vi "AudioIn Block Config Pane.vi"(6 "_SubPanelMessages":refnum<notifier>, 9 "_myEmbeddedToFrameEvent":T7, 10 "_myEmbedded.Exit":refnum<user-event>, 11 "-Property Bundle":cluster{"Name":string, "Value":variant}[](array[cluster])) -> (1 "_Connection Informations":T3, 2 "_Scripter Input":T9)   [LabVIEW 2021]
doc: "Reads values from one or more audio input channels on the NI myRIO. Use this Express VI to read multiple samples for each channel at one time."
uses:
  <vilib>/myRIO/Common/Express VI Framework/xctls/myRIO Channel List/myRIO Channel List.xctl
  <vilib>/myRIO/Common/Express VI Framework/typedefs/Config Pane to Framework Ref.ctl
  <vilib>/myRIO/Common/Express VI Framework/typedefs/Data Validate Ref.ctl
  <vilib>/myRIO/Common/Express VI Framework/typedefs/Scripter Input.ctl
  <vilib>/myRIO/Common/Express VI Framework/typedefs/WireThrough Terminal Names.ctl
  <vilib>/myRIO/Common/Express VI Framework/typedefs/Instrument Driver Method Descriptor Array.ctl
  <vilib>/myRIO/Common/Express VI Framework/typedefs/Instrument Driver Method Descriptor.ctl
  <vilib>/myRIO/Common/Express VI Framework/typedefs/Sub Panel Messages.ctl
  <vilib>/myRIO/Common/Express VI Framework/typedefs/Connection Informations.ctl
  <vilib>/myRIO/Common/Instrument Driver Framework/Utilities/typedefs/Channel Types.ctl
  <vilib>/myRIO/Common/Express VI Framework/vis/Express VI Framework Strings Global.vi
panel:
  in  "Sample Rate Unit":string="kHz"
  out "_learnMoreLatency":string="Gaps exist between sequential n samples acquisitions. Learn more"
  out "_learnMoreFrequency":string="Detailed information about valid sample rates for this Express VI.  Learn more"
  in  "_Validate":bool
  in  "Sample Rate:":dbl=1.0 caption="Sample rate:"
  in  "Samples to Read:":u32=1000 caption="Samples:" min=1 max=10000
  in  "Name:":string="Audio input (n samples)" caption="Node name:"
  in  "Selected Channel List":T1[](xcontrol)=[{"Channel Name"=0, "Channel Alias"="", "Remove Channel"=FALSE, "Index"=0}, {"Channel Name"=1, "Channel Alias"="", "Remove Channel"=FALSE, "Index"=1}]
  in  "_Default Alias String":string
  in  "_VI Default Name (Edit and make value default)":string="Audio input (n samples)"
  in  "_WireThrough Info (Edit and make value default)":T4={"WireThrough Top In"="AudioIn (N Samples) Ref In", "WireThrough Bottom In"="error in (no error)", "WireThrough Top Out"="AudioIn (N Samples) Ref Out", "WireThrough Bottom Out"="error out"}
  in  "_Template Array (Edit and make value default)":T5=[{"Function Name"="Smart Open", "VI Path"=path "<vilib>/myRIO/Instrument Drivers/Onboard IO/AudioIn Block/vis", "Script"=TRUE, "Inputs"=[{"name"="Channel Names", "value"=variant, "Config Pane Only"=TRUE, "Build Array"=FALSE, "Bundle Cluster"=FALSE, "Show Term"=FALSE, "alias"=[], "Required Input"=FALSE}], "Outputs"=[], "VI Class"=enum."Open", "Controls Refs[]"=[], "Inline"=FALSE}, {"Function Name"="Open", "VI Path"=path "<vilib>/myRIO/Instrument Drivers/Onboard IO/AudioIn Block/vis", "Script"=FALSE, "Inputs"=[{"name"="Channel Names", "value"=variant, "Config Pane Only"=TRUE, "Build Array"=FALSE, "Bundle Cluster"=FALSE, "Show Term"=FALSE, "alias"=[], "Required Input"=FALSE}], "Outputs"=[], "VI Class"=enum."Open", "Controls Refs[]"=[], "Inline"=FALSE}, {"Function Name"="Read", "VI Path"=path "<vilib>/myRIO/Instrument Drivers/Onboard IO/AudioIn Block/vis", "Script"=TRUE, "Inputs"=[{"name"="Number of Samples", "value"=variant, "Config Pane Only"=TRUE, "Build Array"=FALSE, "Bundle Cluster"=FALSE, "Show Term"=FALSE, "alias"=[], "Required Input"=TRUE}, {"name"="Sample Rate [Hz]", "value"=variant, "Config Pane Only"=TRUE, "Build Array"=FALSE, "Bundle Cluster"=FALSE, "Show Term"=FALSE, "alias"=[], "Required Input"=FALSE}], "Outputs"=[{"name"="Values", "value"=variant, "Show Term"=TRUE, "Index Array"=TRUE, "Unbundle Cluster"=FALSE, "alias"=[]}], "VI Class"=enum."Data", "Controls Refs[]"=[], "Inline"=FALSE}, {"Function Name"="Close", "VI Path"=path "<vilib>/myRIO/Instrument Drivers/Onboard IO/AudioIn Block/vis", "Script"=FALSE, "Inputs"=[], "Outputs"=[], "VI Class"=enum."Close", "Controls Refs[]"=[], "Inline"=FALSE}]
  in  "_Test Close":bool
  # "User Visible Area"
  # "NOTE: Tab Order has been set\nfor this Front Panel.\n1. Name: (string control)\n2. Add Channel (button)\n3. Selected Channel List (array)\n\nAll other controls are excluded \nfrom Tabbing order\n\nTo exlude a control from context\nhelp prefix its label text with a '-'"
  # "kHz"
  # "Gap:"
  # "Acquired signal"
  # "Missed signal"
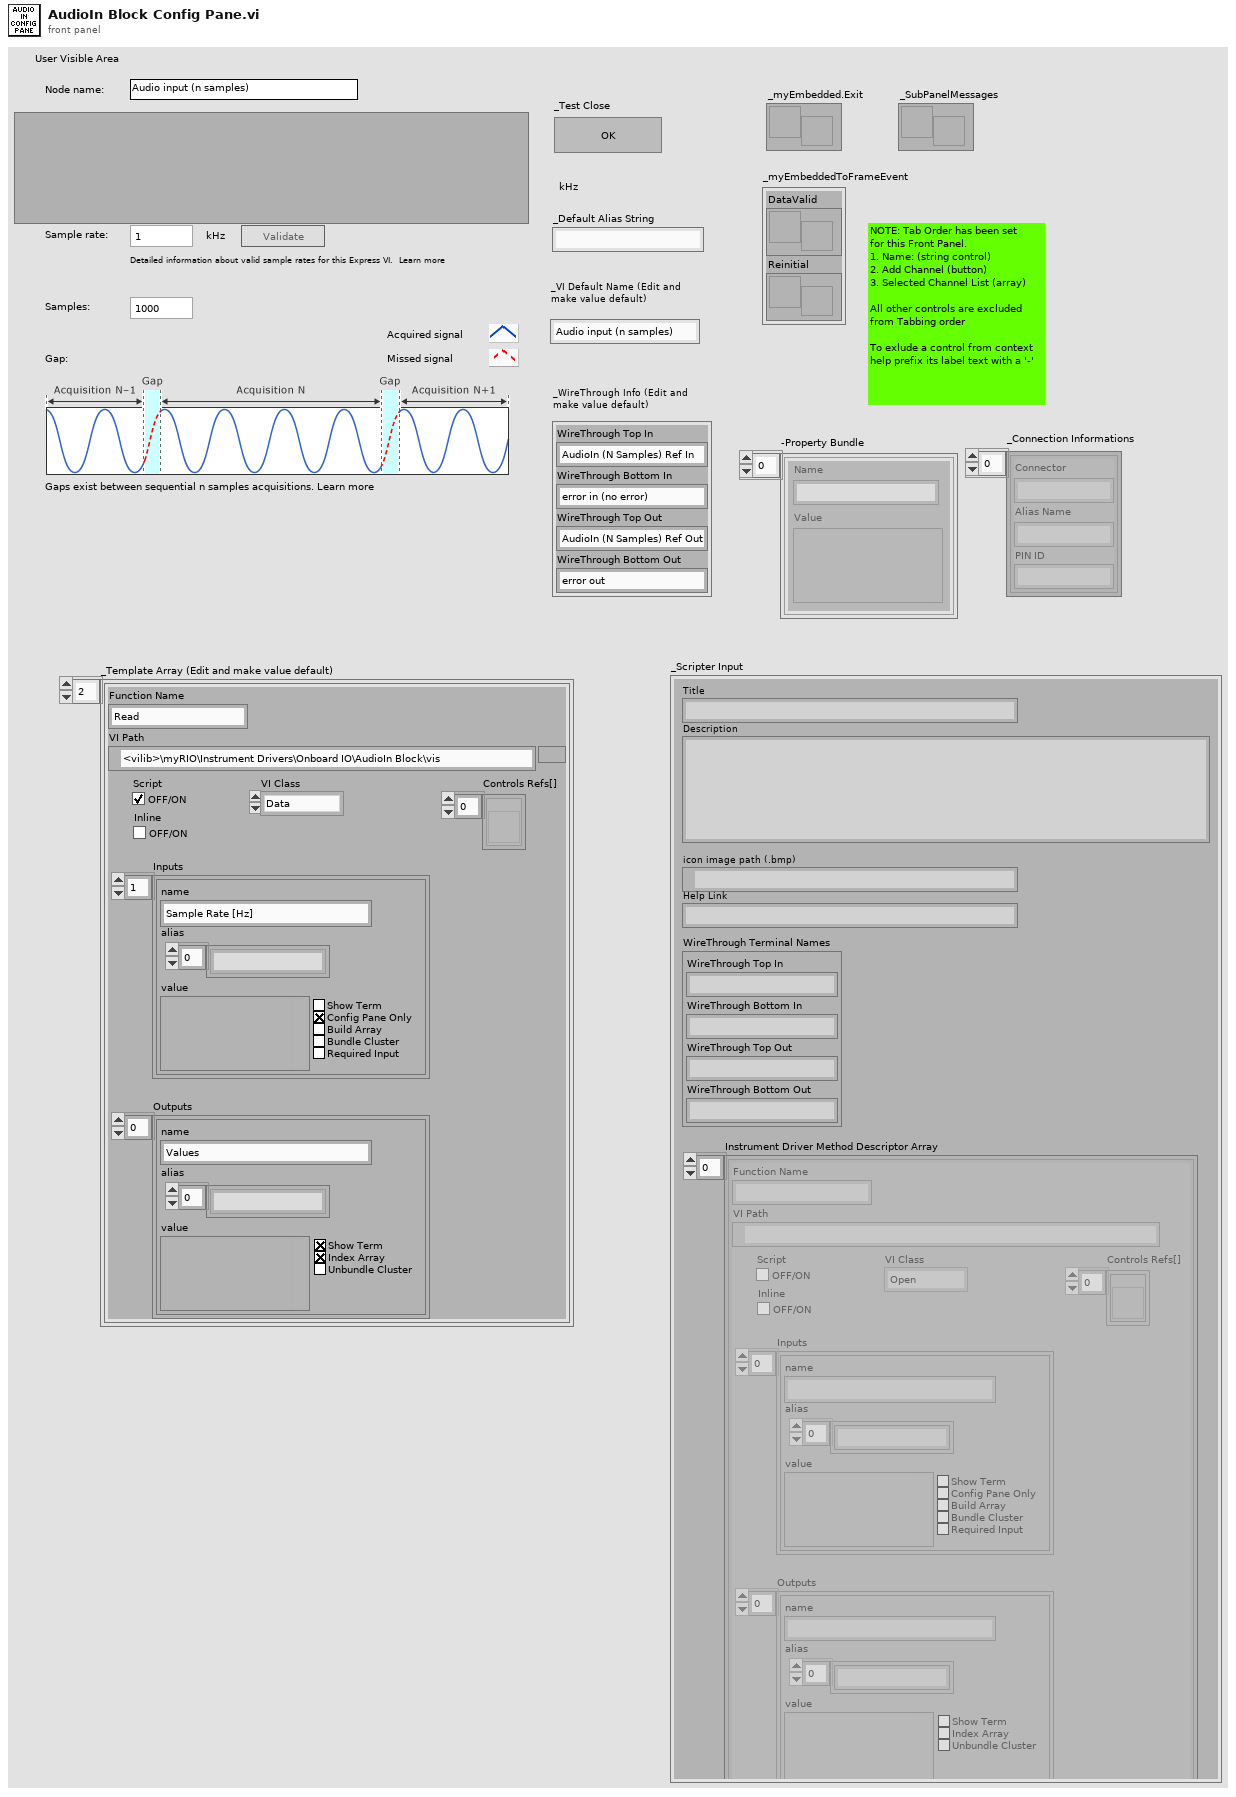
[diagram p1: front panel]
types:
  T1 = typedef "myRIO Channel List.xctl/Channel Data.ctl" = cluster{"Channel Name":u16, "Channel Alias":string, "Remove Channel":T2, "Index":i32}
  T2 = typedef "myRIO Channel List.xctl/Remove Channel.ctl" = bool
  T3 = typedef "Connection Informations.ctl" = cluster{"Connector":string, "Alias Name":string, "PIN ID":string}[]
  T4 = typedef "WireThrough Terminal Names.ctl" = cluster{"WireThrough Top In":string, "WireThrough Bottom In":string, "WireThrough Top Out":string, "WireThrough Bottom Out":string}
  T5 = typedef "Instrument Driver Method Descriptor Array.ctl" = T6[]
  T6 = typedef "Instrument Driver Method Descriptor.ctl" = cluster{"Function Name":string, "VI Path":path, "Script":bool, "Inputs":cluster{"name":string, "value":variant, "Config Pane Only":bool, "Build Array":bool, "Bundle Cluster":bool, "Show Term":bool, "alias":string[], "Required Input":bool}[], "Outputs":cluster{"name":string, "value":variant, "Show Term":bool, "Index Array":bool, "Unbundle Cluster":bool, "alias":string[]}[], "VI Class":enum16{"Open", "Configure", "Data", "Manage", "Close"}, "Controls Refs[]":refnum<vi>[], "Inline":bool}
  T7 = typedef "Config Pane to Framework Ref.ctl" = cluster{"DataValid":T8, "Reinitial":refnum<user-event>}
  T8 = typedef "Data Validate Ref.ctl" = refnum<user-event>
  T9 = typedef "Scripter Input.ctl" = cluster{"Title":string, "Description":string, "icon image path (.bmp)":path, "Help Link":string, "WireThrough Terminal Names":T4, "Instrument Driver Method Descriptor Array":T5}
  T10 = typedef "Channel Types.ctl" = enum32{"Unknown", "AI", "AO", "DIO - DI", "DIO", "DIO - DO", "I2C", "PWM", "Encoder", "SPI", "UART", "Accelerometer", "DIO - LED", "DIO - Button", "AI (N Samples)", "AudioIn (N Samples)", "AO (N Samples)", "AudioOut (N Samples)", "DI (N Samples)", "DO (N Samples)", "AI IRQ", "DI IRQ", "Timer IRQ", "RSL", "Relay", "CAN", "AI (Continuous)", "AO (Continuous)"}
  T11 = typedef "Channel Info.ctl" = cluster{"Channel Name":string, "Alias":string, "Used?":bool, "Not Support?":bool, "Property Bundle":cluster{"Name":string, "Value":variant}[]}
  T12 = typedef "Sub Panel Messages.ctl" = enum16{"Initialized"}
  T13 = enum8{"Enabled", "Disabled", "Disabled and Grayed Out"}
  T14 = cluster{"Connector":string, "Alias Name":string, "PIN ID":string}[]
  T15 = cluster{"name":string, "value":variant, "Config Pane Only":bool, "Build Array":bool, "Bundle Cluster":bool, "Show Term":bool, "alias":string[], "Required Input":bool}[]
  T16 = cluster{"name":string, "value":variant, "Config Pane Only":bool, "Build Array":bool, "Bundle Cluster":bool, "Show Term":bool, "alias":string[], "Required Input":bool}
  T17 = cluster{"name":string, "value":variant, "Show Term":bool, "Index Array":bool, "Unbundle Cluster":bool, "alias":string[]}[]
  T18 = cluster{"name":string, "value":variant, "Show Term":bool, "Index Array":bool, "Unbundle Cluster":bool, "alias":string[]}
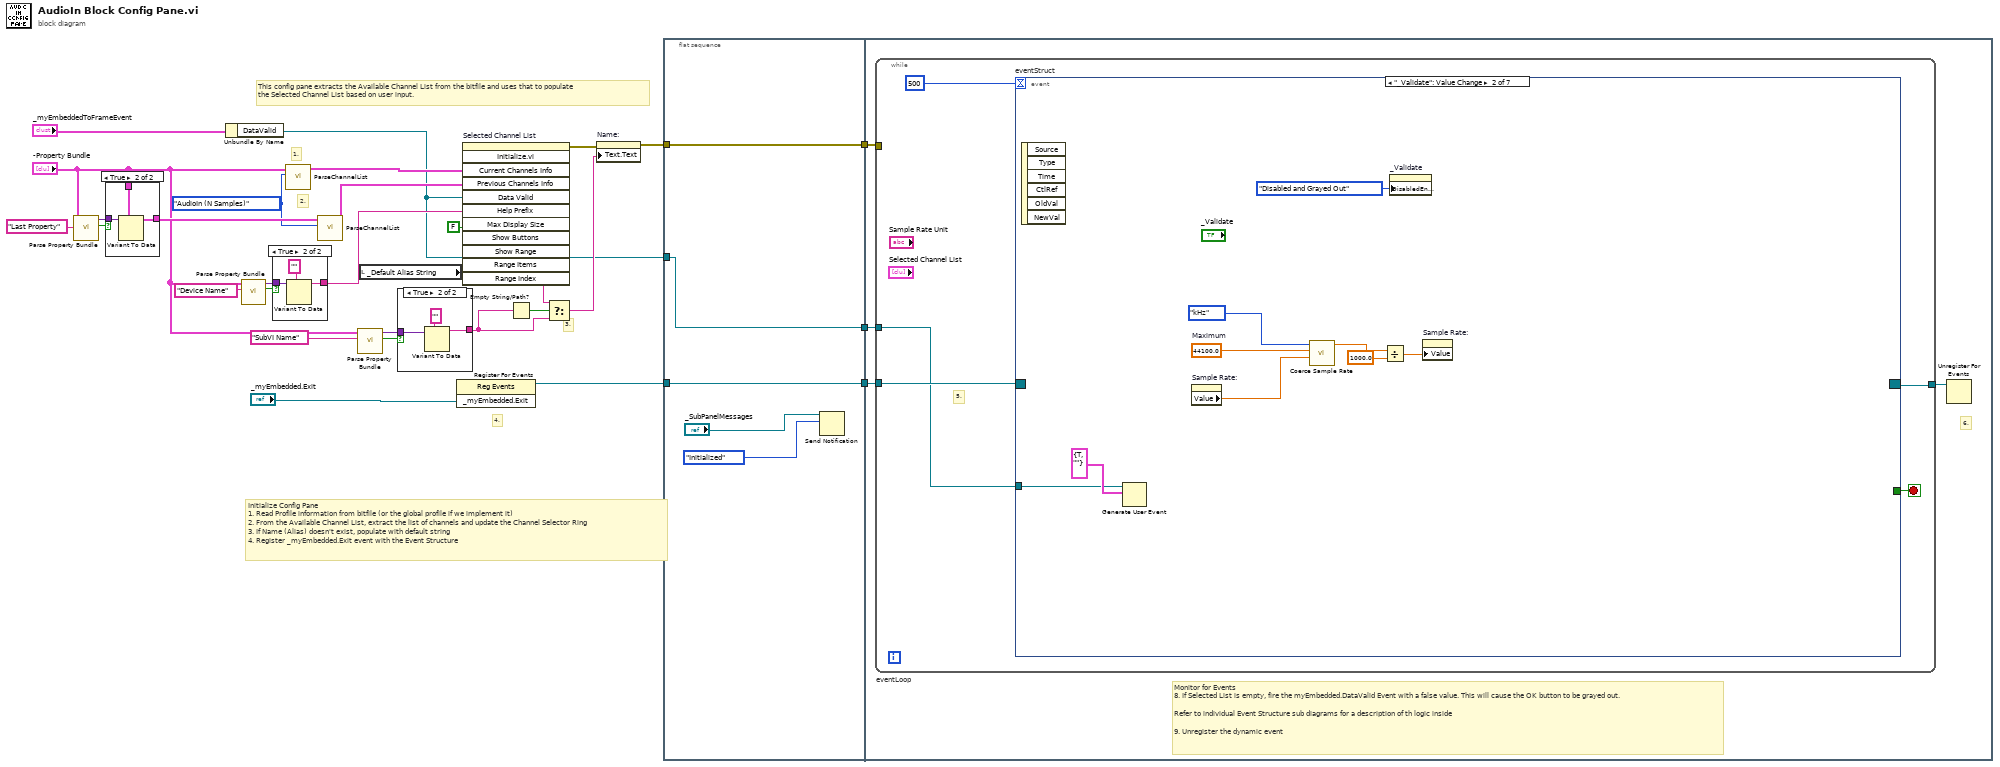
[diagram p0: block diagram]
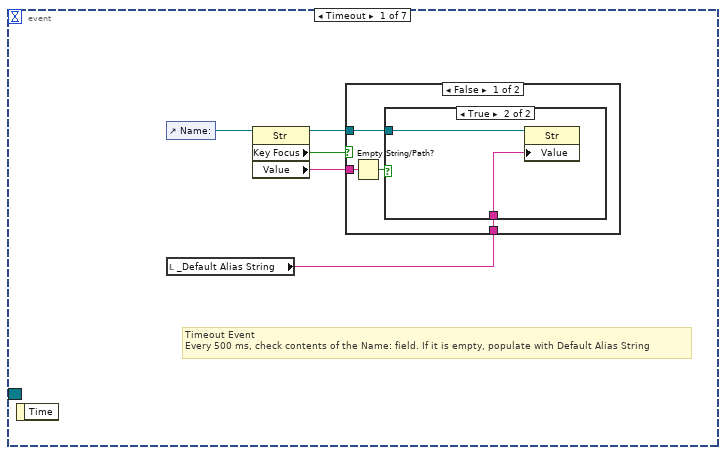
[diagram p2: hidden frame]
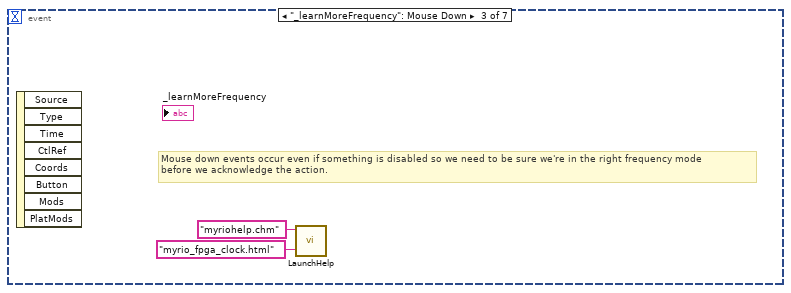
[diagram p5: hidden frame]
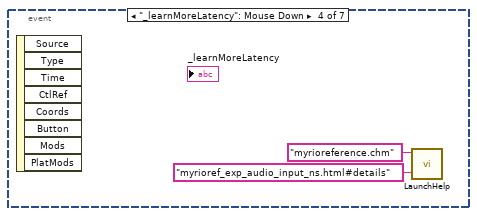
[diagram p6: hidden frame]
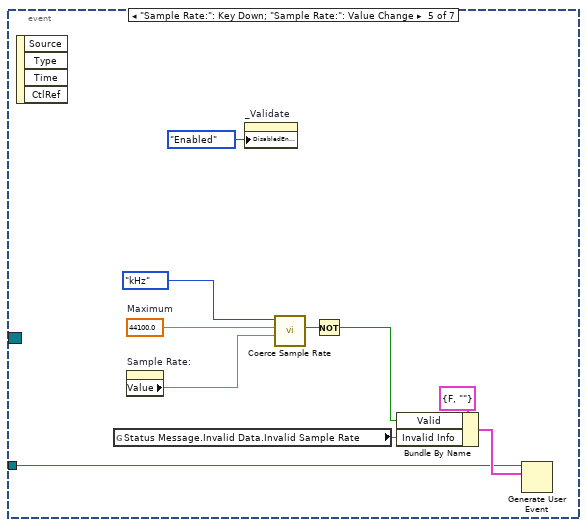
[diagram p7: hidden frame]
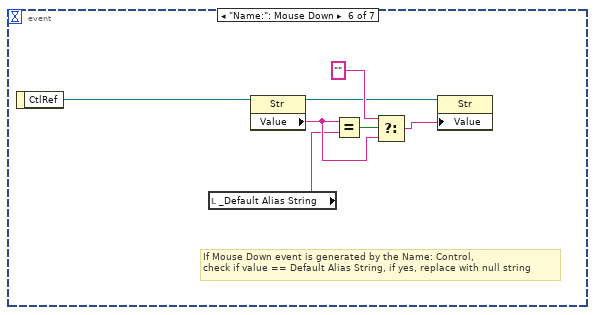
[diagram p8: hidden frame]
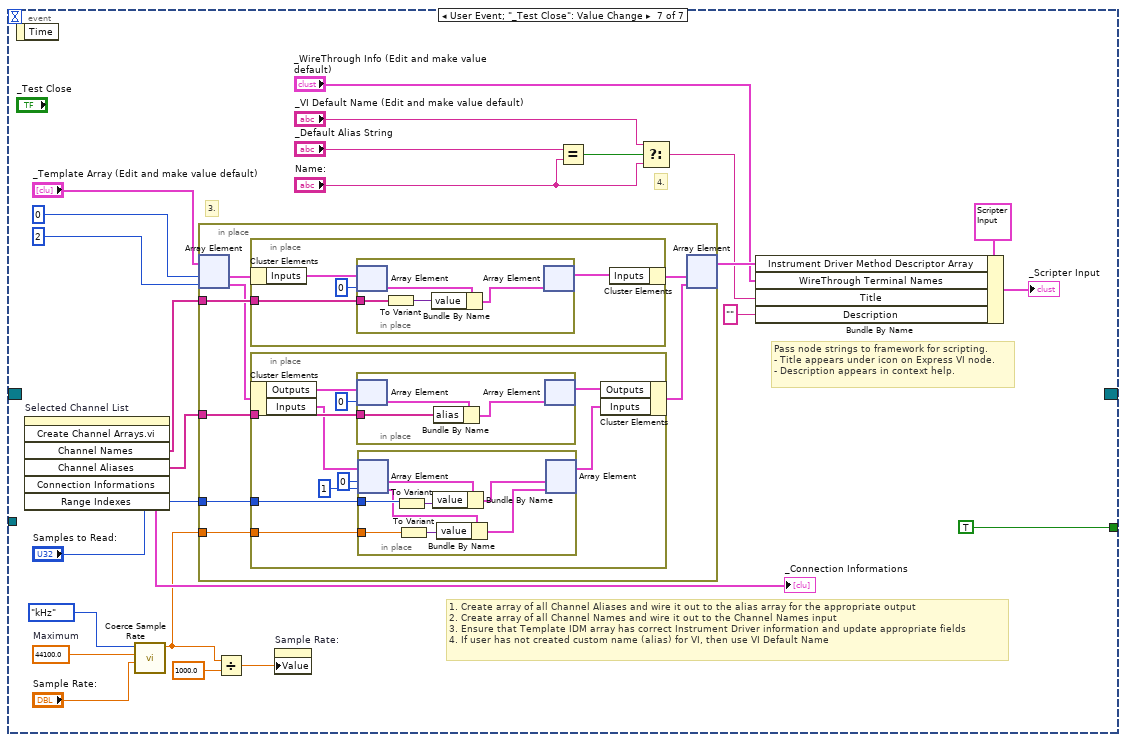
[diagram p9: hidden frame]
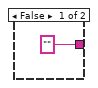
[diagram p12: hidden frame]
diagram:
  w12 = Channel_Types."AudioIn (N Samples)" ("Channel to Read")
  # "2."
  # "1."
  # "This config pane extracts the Available Channel List from the bitfile and uses that to populate\nthe Selected Channel List based on user input."
  # "4."
  # "3."
  # "Initialize Config Pane\n1. Read Profile information from bitfile (or the global profile if we implement it)\n2. From the Available Channel List, extract the list of channels and update the Channel Selector Ring\n3. If Name (Alias) doesn't exist, populate with default string\n4. Register _myEmbedded.Exit event with the Event Structure"
  n1 = call <vilib>:"Parse Property Bundle.vi"("Name"="Last Property", "Property Bundle"="-Property Bundle") -> ("Found?"=w15:bool, "Value"=w16:variant)  [unwired: 8 in]
  n2 = case shown="True" w15 {
    tunnel: w16 -> [_ w32]
    tunnel: [_ w31] -> w14
    tunnel: "-Property Bundle" -> [_ w30]
    frame False {
    }
    frame True {
      n3 = Variant To Data(type=w30, Variant=w32) -> (data=w31:cluster{"Name":string, "Value":variant}[])  [unwired: 1 in, 1 out]
    }
  }
  n4 = Unbundle By Name("_myEmbeddedToFrameEvent") -> ("DataValid"=w2:T8)
  n5 = call <vilib>:"Parse Property Bundle.vi"("Name"="Device Name", "Property Bundle"="-Property Bundle") -> ("Found?"=w9:bool, "Value"=w8:variant)  [unwired: 8 in]
  n6 = case shown="True" w9 {
    tunnel: w8 -> [_ w35]
    tunnel: [_ w34] -> w5
    frame False {
    }
    frame True {
      n7 = Variant To Data(type="", Variant=w35) -> (data=w34:string)  [unwired: 1 in, 1 out]
    }
  }
  n8 = call <vilib>:"ParseChannelList.vi"("Channel to Read"=w12, "_Property Bundle"="-Property Bundle") -> ("Channel List Out"=w19:T11[])  [unwired: 7 in, 2 out]
  n9 = call <vilib>:"ParseChannelList.vi"("Channel to Read"=w12, "_Property Bundle"=w14) -> ("Channel List Out"=w13:T11[])  [unwired: 7 in, 2 out]
  n10 = call <vilib>:"Parse Property Bundle.vi"("Name"="SubVI Name", "Property Bundle"="-Property Bundle") -> ("Found?"=w23:bool, "Value"=w24:variant)  [unwired: 8 in]
  n11 = local read "_Default Alias String"() -> (w18:string)
  n12 = case shown="True" w23 {
    tunnel: w24 -> [_ w39]
    tunnel: ["" ("Name") w37] -> w22
    frame False {
    }
    frame True {
      n13 = Variant To Data(type="" ("Name"), Variant=w39) -> (data=w37:string)  [unwired: 1 in, 1 out]
    }
  }
  n14 = register-events("_myEmbedded.Exit") -> (reference out=w21:refnum<event-registration>)  [unwired: 2 in, 1 out]
  n15 = invoke on="Selected Channel List" class="myRIO Channel List (strict)" method="Initialize.vi"("Current Channels Info"=w19, "Previous Channels Info"=w13, "Data Valid"=w2, "Help Prefix"=w5, "Show Buttons"=FALSE) -> (error out=w20:errorcluster)  [unwired: 7 in, 11 out]
  n16 = Empty String/Path?(string/path=w22) -> (empty?=w28:bool)
  n17 = Select(t=w18, s=w28, f=w22) -> (s? t:f=w27:string)
  n18 = property on="Name:" class="Str"(error in=w20, "Text.Text"=w27) -> (error out=w26:errorcluster)  [unwired: 1 in, 1 out]
  n19 = flat-sequence {
    tunnel: w21 -> [w43]
    tunnel: w26 -> [w44]
    tunnel: [w44] -> w4
    tunnel: [w43] -> w3
    tunnel: w2 -> [w40]
    tunnel: [w40] -> w1
    tunnel: w4 -> [w47]
    tunnel: w3 -> [w46]
    tunnel: w1 -> [w45]
    frame #0 {
      n20 = Send Notification(notification=Sub_Panel_Messages."Initialized", notifier="_SubPanelMessages") -> ()  [unwired: 1 in, 2 out]
    }
    frame #1 {
      # "6."
      # "Monitor for Events\n8. If Selected List is empty, fire the myEmbedded.DataValid Event with a false value. This will cause the OK button to be grayed out.\n\nRefer to individual Event Structure sub diagrams for a description of th logic inside\n\n9. Unregister the dynamic event"
      n21 = while "eventLoop" {
        tunnel: w46 -> [w52]
        tunnel: [w51] -> w48
        tunnel: w47 -> [_]
        tunnel: w45 -> [w49]
        stop <- w53 stop-if-true
        # "5."
        n22 = event "eventStruct" shown="[1] \"_Validate\": Value Change" {
          selector: w52 -> [_ _ _ _ _ _ _]
          dyn-events: [_ _ _ _ _ _ _] -> w51
          timeout: 500 -> [_ _ _ _ _ _ _]
          tunnel: [_ _ _ _ _ _ TRUE ("_Test Close")] -> w53
          tunnel: w49 -> [_ w65 _ _ w80 _ _]
          event Timeout {
            # "Timeout Event\nEvery 500 ms, check contents of the Name: field. If it is empty, populate with Default Alias String"
            n23 = event-data() -> ()  [unwired: 1 in, 1 out]
            n24 = control-ref of="Name:"() -> (w56:refnum<vi>)
            n25 = local read "_Default Alias String"() -> (w54:string)
            n26 = property on="Property Node" class="Str"(reference=w56) -> (reference out=w55:refnum<vi>, "Key Focus"=w57:bool, "Value"=w58:string)  [unwired: 1 in, 1 out]
            n27 = case shown="False" w57 {
              tunnel: w58 -> [w62 _]
              tunnel: w55 -> [w60 _]
              tunnel: w54 -> [w59 _]
              frame False {
                n28 = Empty String/Path?(string/path=w62) -> (empty?=w61:bool)
                n29 = case shown="True" w61 {
                  tunnel: w60 -> [_ w64]
                  tunnel: w59 -> [_ w63]
                  frame False {
                  }
                  frame True {
                    n30 = property on="Property Node" class="Str"(reference=w64, "Value"=w63) -> ()  [unwired: 1 in, 2 out]
                  }
                }
              }
              frame True {
              }
            }
          }
          event "_Validate": Value Change {
            w72 = 44100.0  # Maximum
            n31 = event-data() -> ()  [unwired: 1 in, 6 out]
            n32 = Generate User Event(user event=w65, event data cluster=cluster{"Valid":bool, "Invalid Info":string} {"Valid"=TRUE, "Invalid Info"=""} ("event data")) -> ()  [unwired: 2 in, 2 out]
            n33 = property on="Sample Rate:" class="DigNum (strict)"() -> ("Value"=w71:dbl)  [unwired: 2 in, 2 out]
            n34 = call <vilib>:"Coerce Sample Rate.vi"("Sample Rate:"=w71, "Maximum"=w72, "Sample Rate Unit"=enum16{"Hz", "kHz", "MHz"}."kHz") -> ("Actual Sample Rate (s)"=w69:dbl)  [unwired: 7 in, 1 out]
            n35 = Divide(x=w69, y=1000.0) -> (x/y=w67:dbl)
            n36 = property on="_Validate" class="Bool"("DisabledEnum"=T13."Disabled and Grayed Out" ("Disabled")) -> ()  [unwired: 2 in, 2 out]
            n37 = property on="Sample Rate:" class="DigNum (strict)"("Value"=w67) -> ()  [unwired: 2 in, 2 out]
          }
          event "_learnMoreFrequency": Mouse Down {
            # "Mouse down events occur even if something is disabled so we need to be sure we're in the right frequency mode\nbefore we acknowledge the action."
            n38 = event-data() -> ()  [unwired: 1 in, 8 out]
            n39 = call <vilib>:"LaunchHelp.vi"("Help Topic"="myrio_fpga_clock.html", "Help File"="myriohelp.chm") -> ()  [unwired: 10 in]
          }
          event "_learnMoreLatency": Mouse Down {
            n40 = event-data() -> ()  [unwired: 1 in, 8 out]
            n41 = call <vilib>:"LaunchHelp.vi"("Help Topic"="myrioref_exp_audio_input_ns.html#details", "Help File"="myrioreference.chm") -> ()  [unwired: 10 in]
          }
          event "Sample Rate:": Key Down; "Sample Rate:": Value Change {
            w86 = 44100.0  # Maximum
            n42 = event-data() -> ()  [unwired: 1 in, 4 out]
            n43 = global read "Express VI Framework Strings Global.vi" "Status Message.Invalid Data.Invalid Sample Rate"() -> (w81:string)
            n44 = property on="Sample Rate:" class="DigNum (strict)"() -> ("Value"=w85:dbl)  [unwired: 2 in, 2 out]
            n45 = property on="_Validate" class="Bool"("DisabledEnum"=T13."Enabled" ("Disabled")) -> ()  [unwired: 2 in, 2 out]
            n46 = call <vilib>:"Coerce Sample Rate.vi"("Sample Rate:"=w85, "Maximum"=w86, "Sample Rate Unit"=enum16{"Hz", "kHz", "MHz"}."kHz") -> ("Coercion needed?"=w79:bool)  [unwired: 7 in, 1 out]
            n47 = Not(x=w79) -> (.not. x?=w78:bool)
            n48 = Bundle By Name(cluster=cluster{"Valid":bool, "Invalid Info":string} {"Valid"=FALSE, "Invalid Info"=""} ("event data"), "Valid"=w78, "Invalid Info"=w81) -> (w82:cluster{"Valid":bool, "Invalid Info":string})
            n49 = Generate User Event(user event=w80, event data cluster=w82) -> ()  [unwired: 2 in, 2 out]
          }
          event "Name:": Mouse Down {
            # "If Mouse Down event is generated by the Name: Control,\ncheck if value == Default Alias String, if yes, replace with null string"
            n50 = event-data() -> ("CtlRef"=w94:refnum<vi>)  [unwired: 1 in]
            n51 = local read "_Default Alias String"() -> (w88:string)
            n52 = property class="Str"(reference=w94) -> (reference out=w90:refnum<vi>, "Value"=w89:string)  [unwired: 1 in, 1 out]
            n53 = Equal?(x=w89, y=w88) -> (x = y?=w93:bool)
            n54 = Select(t="", s=w93, f=w89) -> (s? t:f=w91:string)
            n55 = property class="Str"(reference=w90, "Value"=w91) -> ()  [unwired: 1 in, 2 out]
          }
          event User Event; "_Test Close": Value Change {
            w103 = 44100.0  # Maximum
            # "1. Create array of all Channel Aliases and wire it out to the alias array for the appropriate output\n2. Create array of all Channel Names and wire it out to the Channel Names input\n3. Ensure that Template IDM array has correct Instrument Driver information and update appropriate fields\n4. If user has not created custom name (alias) for VI, then use VI Default Name"
            # "4."
            # "3."
            # "Pass node strings to framework for scripting.\n- Title appears under icon on Express VI node.\n- Description appears in context help."
            n56 = event-data() -> ()  [unwired: 1 in, 1 out]
            n57 = invoke on="Selected Channel List" class="myRIO Channel List (strict)" method="Create Channel Arrays.vi"() -> ("Channel Names"=w101:string[], "Channel Aliases"=w100:string[], "Connection Informations"=→"_Connection Informations":T14)  [unwired: 7 in, 4 out]
            n58 = call <vilib>:"Coerce Sample Rate.vi"("Sample Rate:"="Sample Rate:", "Maximum"=w103, "Sample Rate Unit"=enum16{"Hz", "kHz", "MHz"}."kHz") -> ("Actual Sample Rate (s)"=w97:dbl)  [unwired: 7 in, 1 out]
            n59 = in-place {
              in-place-border: w101 -> [w123]
              in-place-border: w100 -> [w122]
              in-place-border: "Samples to Read:" -> [w120]
              in-place-border: w97 -> [w119]
              n60 = in-place-array #1("_Template Array (Edit and make value default)", 0, 2) -> (w126:T6, w121:T6)
              n61 = in-place {
                in-place-border: w123 -> [w150]
                n62 = in-place-cluster #2(w126) -> ("Inputs"=w151:T15)
                n63 = in-place {
                  in-place-border: w150 -> [w152]
                  n64 = in-place-array #3(w151, 0) -> (w155:T16)
                  n65 = To Variant(anything=w152) -> (Variant=w153:variant)
                  n66 = Bundle By Name(cluster=w155, "value"=w153) -> (w154:T16)
                  n67 = in-place-array #3(w154) -> (w149:T15)  [unwired: 1 out]
                }
                n68 = in-place-cluster #2("Inputs"=w149) -> (w125:T6)
              }
              n69 = in-place {
                in-place-border: w122 -> [w135]
                in-place-border: w120 -> [w129]
                in-place-border: w119 -> [w128]
                n70 = in-place-cluster #4(w121) -> ("Outputs"=w136:T17, "Inputs"=w132:T15)
                n71 = in-place {
                  in-place-border: w135 -> [w145]
                  n72 = in-place-array #5(w136, 0) -> (w147:T18)
                  n73 = Bundle By Name(cluster=w147, "alias"=w145) -> (w146:T18)
                  n74 = in-place-array #5(w146) -> (w134:T17)  [unwired: 1 out]
                }
                n75 = in-place {
                  in-place-border: w129 -> [w142]
                  in-place-border: w128 -> [w139]
                  n76 = in-place-array #6(w132, 0, 1) -> (w144:T16, w140:T16)
                  n77 = To Variant(anything=w142) -> (Variant=w141:variant)
                  n78 = To Variant(anything=w139) -> (Variant=w138:variant)
                  n79 = Bundle By Name(cluster=w144, "value"=w141) -> (w143:T16)
                  n80 = Bundle By Name(cluster=w140, "value"=w138) -> (w137:T16)
                  n81 = in-place-array #6(w143, w137) -> (w131:T15)  [unwired: 2 out]
                }
                n82 = in-place-cluster #4("Outputs"=w134, "Inputs"=w131) -> (w124:T6)
              }
              n83 = in-place-array #1(w125, w124) -> (w116:T5)  [unwired: 2 out]
            }
            n84 = Divide(x=w97, y=1000.0) -> (x/y=w95:dbl)
            n85 = property on="Sample Rate:" class="DigNum (strict)"("Value"=w95) -> ()  [unwired: 2 in, 2 out]
            n86 = Equal?(x="_Default Alias String", y="Name:") -> (x = y?=w108:bool)
            n87 = Select(t="_VI Default Name (Edit and make value default)", s=w108, f="Name:") -> (s? t:f=w106:string)
            n88 = Bundle By Name(cluster=T9 {"Title"="", "Description"="", "icon image path (.bmp)"=path "", "Help Link"="", "WireThrough Terminal Names"={"WireThrough Top In"="", "WireThrough Bottom In"="", "WireThrough Top Out"="", "WireThrough Bottom Out"=""}, "Instrument Driver Method Descriptor Array"=[]} ("Scripter Input"), "Instrument Driver Method Descriptor Array"=w116, "WireThrough Terminal Names"="_WireThrough Info (Edit and make value default)", "Title"=w106, "Description"="" ("Title")) -> (→"_Scripter Input":T9)
          }
        }
      }
      n89 = Unregister For Events(event registration refnum=w48) -> ()  [unwired: 1 in, 1 out]
    }
  }
